vi "Destroy BrowerGuidencer.vi"(0 "reference in":refnum<class "BrowerGuidencer.lvclass">, 5 "error in (no error)":errorcluster) -> (14 "reference out":refnum<class "BrowerGuidencer.lvclass">, 19 "error out":errorcluster)   [LabVIEW 2015, in "BrowerGuidencer.lvclass"]
uses:
  BrowerGuidencer.lvclass
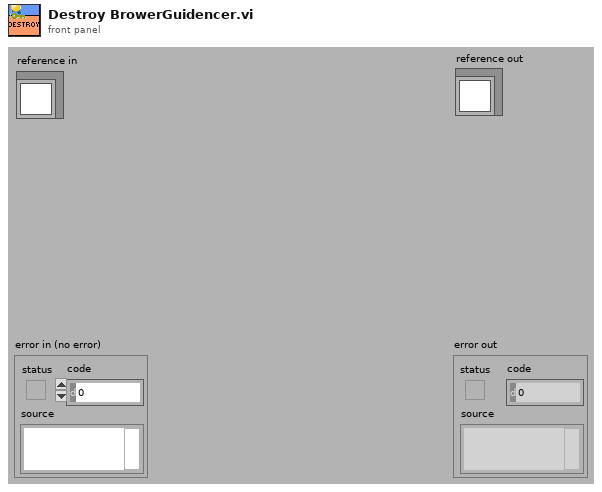
[diagram p1: front panel]
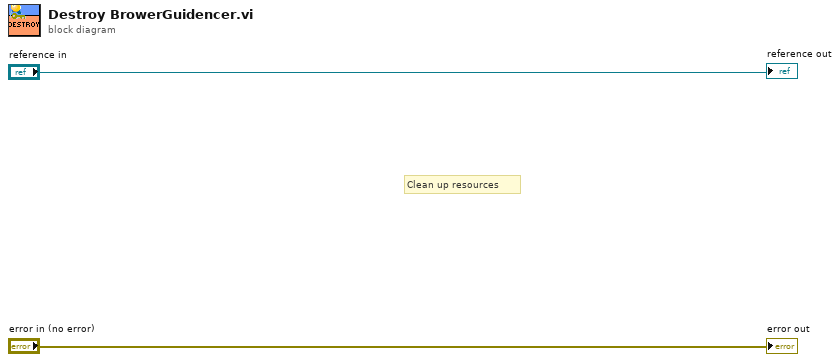
[diagram p0: block diagram]
diagram:
  # "Clean up resources"
  "error out" <- "error in (no error)"
  "reference out" <- "reference in"
